vi "退出系统对话框.vi"(1 "退出":bool, 2 "error in (no error)":errorcluster) -> (0 "T/F":bool)   [LabVIEW 2019]
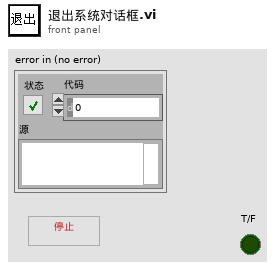
[diagram p1: front panel]
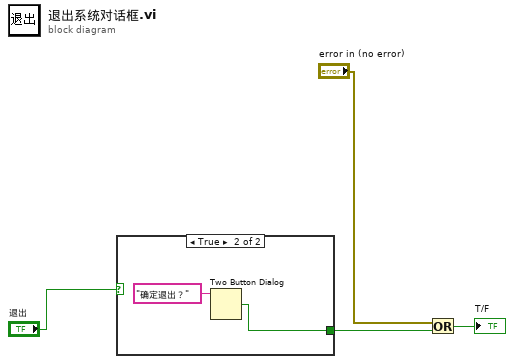
[diagram p0: block diagram]
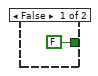
[diagram p2: hidden frame]
diagram:
  n1 = case shown="True" "退出" {
    tunnel: [FALSE ("T button?") w6] -> w3
    frame False {
    }
    frame True {
      n2 = Two Button Dialog(message="确定退出？" ("消息")) -> (T button?=w6:bool)  [unwired: 2 in]
    }
  }
  n3 = Or(x="error in (no error)", y=w3) -> (x .or. y?=→"T/F":bool)
